vi "qrcode.vi"() -> ()   [LabVIEW 2021]
panel:
  out "qrcode":picture
  out "error out":errorcluster
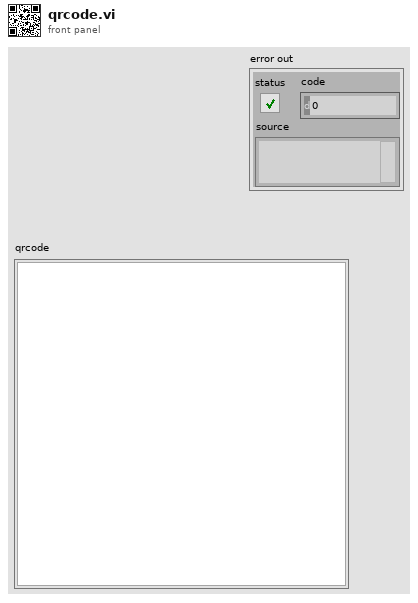
[diagram p1: front panel]
types:
  T1 = typedef "imagedata.ctl" = cluster{"image type":i32, "image depth":i32, "image":u8[], "mask":u8[], "colors":u32[], "Rectangle":cluster{"left":i16, "top":i16, "right":i16, "bottom":i16}}
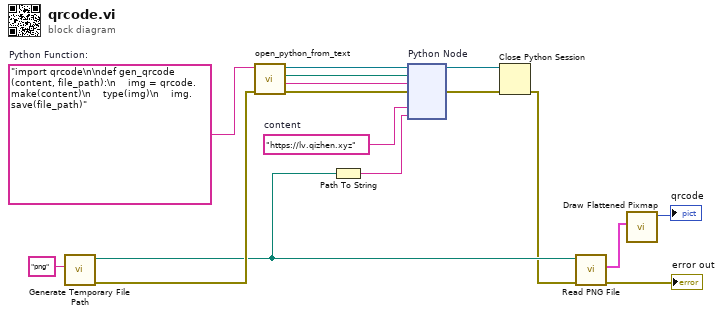
[diagram p0: block diagram]
diagram:
  w8 = "https://lv.qizhen.xyz"  # content
  w12 = "import qrcode\n\ndef gen_qrcode (content, file_path):\n    img = qrcode.make(content)\n    type(img)\n    img.save(file_path)"  # Python Function:
  n1 = call <vilib>:"Generate Temporary File Path.vi"("Temporary File Extension (tmp)"="png") -> ("error out"=w4:errorcluster, "Unique Temporary File Path"=w3:path)  [unwired: 9 in]
  n2 = call "open_python_from_text.vi"("error in (no error)"=w4, "Python Function:"=w12) -> ("error out"=w14:errorcluster, "function name"=w10:string, "module path"=w11:path, "Refnum out"=w16:refnum<k35>)  [unwired: 6 in]
  n3 = Path To String(path=w3) -> (string=w7:string)
  n4 = node "Python Node"(w16, w11, w10, w14, w8, w7) -> (w15:refnum<k35>, w13:errorcluster)  [unwired: 4 in, 2 out]
  n5 = Close Python Session(session in=w15, error in=w13) -> (11:w2:errorcluster)
  n6 = call <vilib>:"Read PNG File.vi"("error in (no error)"=w2, "path to PNG file"=w3) -> ("error out"=→"error out":errorcluster, "image data"=w5:T1)  [unwired: 7 in, 1 out]
  n7 = call <vilib>:"Draw Flattened Pixmap.vi"("image data"=w5) -> ("new picture"=→"qrcode":picture)  [unwired: 8 in]
